vi "RS232_W.vi"(8 "error in (no error)":errorcluster caption="错误输入（无错误）", 10 "CMD":string, 11 "VISA资源名称":refnum<visa-resource-name>) -> (0 "error out":errorcluster caption="错误输出", 1 "CMD 2":string, 3 "VISA资源名称输出":refnum<visa-resource-name>)   [LabVIEW 2018]
panel:
  # "opena-01-02"
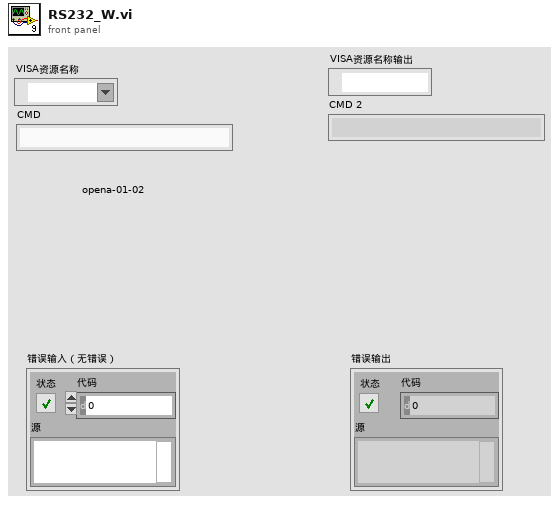
[diagram p1: front panel]
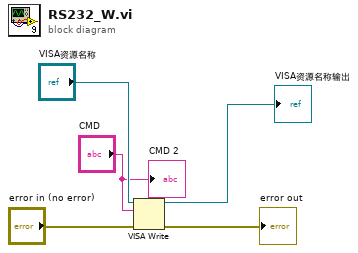
[diagram p0: block diagram]
diagram:
  n1 = VISA Write(VISA resource name="VISA资源名称", write buffer="CMD", error in (no error)="error in (no error)") -> (VISA resource name out=→"VISA资源名称输出":refnum<visa-resource-name>, error out=→"error out":errorcluster)  [unwired: 1 out]
  "CMD 2" <- "CMD"
